vi "Start VST.vi"(8 "error in (no error)":errorcluster, 10 "VST Config":T1={"Samples to Read per Block"=33554432, "IQ rate (S/s)"=1250000000.0, "Carrier Frequency (Hz)"=1000000000.0, "Reference Level (dBm)"=0.0, "Resource Name"="RFSA", "Clock Source"="OnboardClock", "Host DMA Buffer Size"=2000000000} {"Host DMA Buffer Size" format="%.0p"; "Reference Level (dBm)" format="%.2f"; "Carrier Frequency (Hz)" format="%#.3p"; "IQ rate (S/s)" format="%#.3p"; "Samples to Read per Block" min=1 format="%.0p"}, 11 "Application Manager in":refnum<class "Application Manager.lvclass">) -> (0 "error out":errorcluster, 3 "Application Manager out":refnum<class "Application Manager.lvclass">)   [LabVIEW 2020, in "Application Manager.lvlib" / "Application Manager.lvclass"]
uses:
  Application Manager.lvclass
  RFSA DAQ/RFSA DAQ/Configure VST.ctl
  Signal Analysis/Signal Analysis/Low Prio Rendering.ctl
  Application Manager.lvclass/Application Manager.ctl
  Signal Analysis/Signal Analysis Messages/Set Render Prio Msg/Set Render Prio Msg.lvclass/Set Render Prio Msg.ctl
  <vilib>/ActorFramework/Message Enqueuer/Message Enqueuer.lvclass/Message Enqueuer.ctl
  RFSA DAQ/RFSA DAQ Messages/Configure VST Msg/Configure VST Msg.lvclass/Configure VST Msg.ctl
  <vilib>/ActorFramework/Message Enqueuer/Enqueue.vi
  Signal Analysis/Signal Analysis Messages/Set Render Prio Msg/Set Render Prio Msg.lvclass
  C:/Program Files/National Instruments/LabVIEW 2025/vi.lib/ActorFramework/Message/Message.lvclass
  RFSA DAQ/RFSA DAQ Messages/Configure VST Msg/Configure VST Msg.lvclass
  DAQ Interface/DAQ Interface Messages/Start DAQ Msg/Start DAQ Msg.lvclass
  <vilib>/ActorFramework/Message Priority Queue/Priority Enqueue.vi
  Signal Analysis/Signal Analysis/Signal Analysis.lvclass
  RFSA DAQ/RFSA DAQ/RFSA DAQ.lvclass
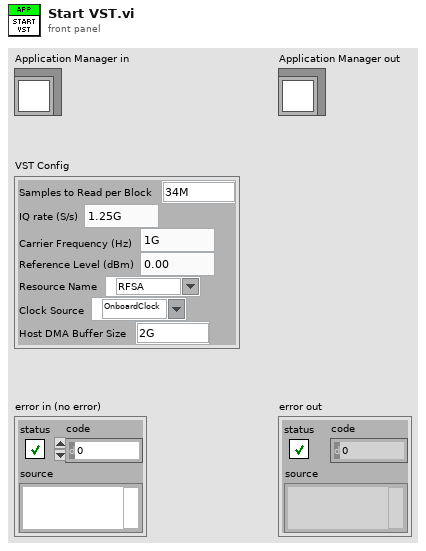
[diagram p1: front panel]
types:
  T1 = typedef "RFSA DAQ.lvlib/RFSA DAQ.lvclass/Configure VST.ctl" = cluster{"Samples to Read per Block":i32, "IQ rate (S/s)":dbl, "Carrier Frequency (Hz)":dbl, "Reference Level (dBm)":dbl, "Resource Name":refnum<k15>, "Clock Source":refnum<k15>, "Host DMA Buffer Size":i64}
  T2 = typedef "Signal Analysis.lvlib/Signal Analysis.lvclass/Low Prio Rendering.ctl" = cluster{"Low Prio Rendering":bool}
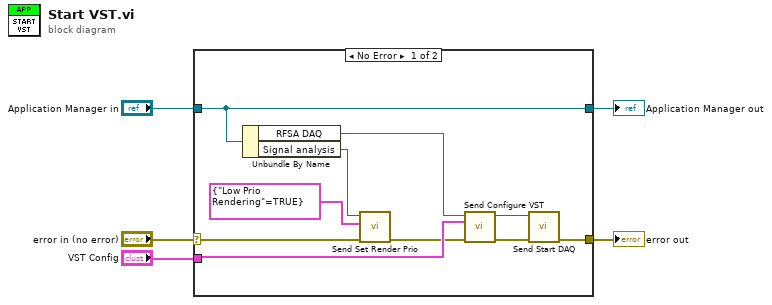
[diagram p0: block diagram]
diagram:
  n1 = case shown="No Error" "error in (no error)" {
    selector: "error in (no error)" -> [w7 w17]
    tunnel: [w10 w17] -> w4
    tunnel: [w15 w16] -> w2
    tunnel: "Application Manager in" -> [w15 w16]
    tunnel: "VST Config" -> [w13 _]
    frame No Error {
      n2 = Unbundle By Name(w15) -> ("RFSA DAQ"=w14:refnum<class "Message Enqueuer.lvclass">, "Signal analysis"=w9:refnum<class "Message Enqueuer.lvclass">)
      n3 = call "Send Set Render Prio.vi"("error in (no error)"=w7, "Low Prio Rendering"=T2 {"Low Prio Rendering"=TRUE}, "Message Enqueuer"=w9) -> ("error out"=w6:errorcluster)  [unwired: 7 in, 1 out]
      n4 = call "Send Configure VST.vi"("error in (no error)"=w6, "VST Config"=w13, "Message Enqueuer"=w14) -> ("error out"=w11:errorcluster, "Message Enqueuer out"=w12:refnum<class "Message Enqueuer.lvclass">)  [unwired: 7 in]
      n5 = call "Send Start DAQ.vi"("error in (no error)"=w11, "Message Enqueuer"=w12) -> ("error out"=w10:errorcluster)  [unwired: 8 in, 1 out]
    }
    frame Error {
    }
  }
  "error out" <- w4
  "Application Manager out" <- w2
